vi "Call Chain To Hash Hierarchy.vi"(11 "VI Call Chain":string[](array[string])) -> (3 "Flat Hierarchy":string[](array[string]))   [LabVIEW 2013, in "Caraya.lvlib"]
uses:
  Caraya.lvlib
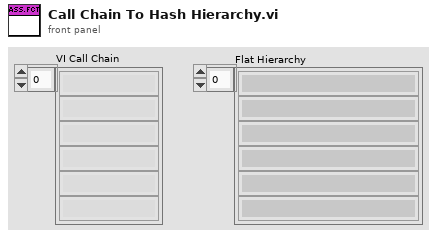
[diagram p1: front panel]
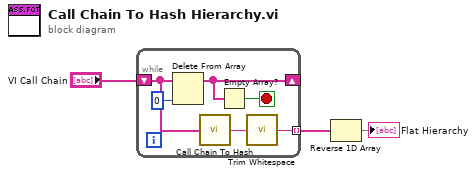
[diagram p0: block diagram]
diagram:
  n1 = while {
    tunnel: [w4] -> w2 mode=indexing
    shift-right: [w7] -> _
    shift-left: "VI Call Chain" -> [w8]
    stop <- w6 stop-if-true
    n2 = Delete From Array(array=w8, index=0) -> (array with subset deleted=w7:string[])  [unwired: 1 in, 1 out]
    n3 = call "Call Chain To Hash.vi"("VI Call Chain"=w8) -> ("Key"=w5:string)
    n4 = Empty Array?(array=w7) -> (empty?=w6:bool)
    n5 = call <vilib>:"Trim Whitespace.vi"("string"=w5) -> ("trimmed string"=w4:string)  [unwired: 1 in]
  }
  n6 = Reverse 1D Array(array=w2) -> (reversed array=→"Flat Hierarchy":string[])
